vi "iscan.vi"(0 "IP adress":string="192.109.209.229", 1 "stop":bool, 2 "Channel":u8(ring)=12 items=["1", "2", "3", "4", "5", "6", "7", "8", "9", "10", "11", "12", "13", "14", "15", "16"], 3 "ISCAN Parameters":T1={"vs_initial "=TRUE, "Current_step"=0.0, "Scans"=[{" vs_initial"=FALSE, "Current_step"=0.001, "Scan_Rate"=1.0}, {" vs_initial"=FALSE, "Current_step"=-0.001, "Scan_Rate"=1.0}, {" vs_initial"=FALSE, "Current_step"=0.0, "Scan_Rate"=1.0}], "Scan_number"=2, "N_Cycles"=1, "Record_every_dI"=1e-05, "Begin_measuring_E"=0.5, "End_measuring_E"=0.75, "I_Range"=7, "E_Range"=2, "Bandwidth"=5, "em"=1, "ce"=0, "tb"=5e-05} {"tb" min=5e-05 max=1 format="%^_3e"; "ce" items=["Standard", "CE to ground"]; "End_measuring_E" min=0 max=1 format="%.2f"; "Begin_measuring_E" min=0 max=1 format="%.2f"; "Current_step" min=-150 max=150 format="%^_3e"; "N_Cycles" min=0 max=1000000; "Scan_number" min=0 max=98; "Scans"."Scan_Rate" min=0.01 max=1000 format="%^_3e"; "Scans"."Current_step" min=-150 max=150 format="%^_3e"; "E_Range" items=["±2.5V", "±5V", "±10V", "Auto"]; "Bandwidth" items=["1"=1, "2"=2, "3"=3, "4"=4, "5"=5, "6"=6, "7"=7, "8"=8, "9"=9]; "Record_every_dI" format="%^_3e"; "I_Range" items=["1pA", "1nA", "10nA", "100nA", "1µA", "10µA", "100µA", "1mA", "10mA", "100mA", "1A", "Booster"]}, 4 "Exit":bool, 5 "Start":bool, 6 "Draw":enum16{"I(Ewe)", "Ewe(t)", "I(t)"}(ring)=enum."I(t)") -> (7 "XY Graph":cluster{"Data 101":sgl[], "Data 101":sgl[]}(graph), 8 "Number of points":i32=105)   [LabVIEW 2016]
doc: "The Current scan technique (Galvanodynamic Technique) technique allows the user to perform galvanodynamic periods with different scan rates.\nIn general, in this VI, the first thing to do is to start by establishing the connection with the instrument defined by its IP adress, then load the firmware in the channel selected, get the information on the plugged channels, load protocol on a channel, start/stop the protocol, retreive data and draw the graph."
uses:
  LLB/dll_Functions.llb/ISCANParameters.ctl
panel:
  in  "Display Parameters?":bool caption="Display Parameters"
  out "DllPath":path caption="DLL Path"
  out "LibVersion":string caption="DLL Version"
  out "Device Code":i32
  out "Exit 2":bool=TRUE
  out "Data 125":sgl[][](array[numeric])=[[0.003, 0.0019739384, 6.01559e-07, 0.002076381], [0.105000004, 0.012167796, 2.1901733e-06, 0.0117511805], [0.20700002, 0.022361653, 3.975648e-06, 0.021977918], [0.30900002, 0.03255551, 5.772186e-06, 0.032090176], [0.411, 0.042749364, 7.5965745e-06, 0.042278755], [0.513, 0.052943222, 9.43279e-06, 0.052619968], [0.615, 0.06313708, 1.1011484e-05, 0.06277039], [0.717, 0.07333094, 1.3262951e-05, 0.07292081], [0.81900007, 0.08352479, 1.5135982e-05, 0.082956746], [0.92, 0.09371865, 1.6970866e-05, 0.09329796], [1.146, 0.08352479, 1.50444275e-05, 0.083796255], [1.248, 0.07333094, 1.3190472e-05, 0.07337872], [1.35, 0.06313708, 1.1359403e-05, 0.06338094], [1.4510001, 0.052943222, 9.505447e-06, 0.053039722], [1.5530001, 0.042749364, 7.704897e-06, 0.042965624], [1.6550001, 0.03255551, 5.7821057e-06, 0.03273889], [1.7570001, 0.022361653, 3.9939605e-06, 0.02243583], [1.8590001, 0.012167796, 2.2004742e-06, 0.012209094], [1.9610001, 0.0019739384, 3.9210917e-07, 0.0019060377], [2.0630002, -0.008219917, -1.42999e-06, -0.007939104], [2.1650002, -0.018413773, -3.2925293e-06, -0.01812768], [2.2670002, -0.02860763, -5.1661327e-06, -0.028087301], [2.3690002, -0.038801484, -7.0229494e-06, -0.038695633], [2.4710002, -0.048995342, -8.872135e-06, -0.048960526], [2.5730002, -0.059189197, -1.0682789e-05, -0.059149105], [2.6750002, -0.069383055, -1.2368184e-05, -0.06929952], [2.7770002, -0.07957691, -1.4145845e-05, -0.079564415], [2.8790002, -0.089770764, -1.595784e-05, -0.08963852], [2.9810002, -0.09996462, -1.7746945e-05, -0.09997973], [3.0830002, -0.11015848, -1.9597086e-05, -0.11005383], [3.1840003, -0.120352335, -2.1420525e-05, -0.1202424], [3.2860003, -0.13054618, -2.3339331e-05, -0.13024017], [3.3880002, -0.14074004, -2.5181842e-05, -0.14054324], [3.4900002, -0.1509339, -2.7039614e-05, -0.15061733], [3.5920002, -0.16112776, -2.8866867e-05, -0.16069143], [3.6940002, -0.17132162, -3.0690302e-05, -0.17118528], [3.7960002, -0.18151547, -3.246415e-05, -0.18129754], [3.8980002, -0.19170932, -3.425326e-05, -0.19167691], [4.1660004, -0.18151547, -3.2410746e-05, -0.1819081], [4.268, -0.17132162, -3.064834e-05, -0.17160504], [4.3700004, -0.16112776, -2.8840164e-05, -0.1615691], [4.472, -0.1509339, -2.6993837e-05, -0.15141869], [4.5740004, -0.14074004, -2.5170399e-05, -0.14126827], [4.676, -0.13054618, -2.3297369e-05, -0.13085073], [4.7780004, -0.120352335, -2.1454858e-05, -0.120471366], [4.88, -0.11015848, -1.9608531e-05, -0.11066438], [4.9820004, -0.09996462, -1.7731685e-05, -0.100361325], [5.084, -0.089770764, -1.5908246e-05, -0.09028722], [5.1860003, -0.07957691, -1.4138216e-05, -0.07979337], [5.288, -0.069383055, -1.23643695e-05, -0.06975743], [5.3900003, -0.059189197, -1.0510413e-05, -0.059530698], [5.491, -0.048995342, -8.728937e-06, -0.049342122], [5.5930004, -0.038801484, -6.897869e-06, -0.039191704], [5.695, -0.02860763, -5.1615543e-06, -0.029041288], [5.7970004, -0.018413773, -3.292148e-06, -0.018547434], [5.899, -0.008219917, -1.4265564e-06, -0.008549656], [6.0010004, 0.0019739384, 4.397981e-07, 0.0014481241], [6.103, 0.012167796, 2.245111e-06, 0.011636702], [6.2050004, 0.022361653, 4.0595805e-06, 0.021939758], [6.307, 0.03255551, 5.846962e-06, 0.032090176], [6.4090004, 0.042749364, 7.638159e-06, 0.04212612], [6.511, 0.052943222, 9.431646e-06, 0.05246733], [6.6130004, 0.06313708, 1.1045057e-05, 0.062579595], [6.715, 0.07333094, 1.3209546e-05, 0.07276817], [6.8170004, 0.08352479, 1.5067316e-05, 0.08303307], [6.919, 0.09371865, 1.690983e-05, 0.09318349], [7.1440005, 0.08352479, 1.5128351e-05, 0.08364362], [7.2460003, 0.07333094, 1.3301099e-05, 0.0733024], [7.3480005, 0.06313708, 1.1408995e-05, 0.06338094], [7.4490004, 0.052943222, 9.520706e-06, 0.053039726], [7.5510006, 0.042749364, 7.704897e-06, 0.042316914], [7.6530004, 0.03255551, 5.7290754e-06, 0.032624412], [7.7550006, 0.022361653, 3.9203287e-06, 0.02262663], [7.8570004, 0.012167796, 2.1073854e-06, 0.012056456], [7.9590006, 0.0019739384, 3.3221184e-07, 0.0022876323], [8.061001, -0.008219917, -1.4410538e-06, -0.007900944], [8.163, -0.018413773, -3.2478924e-06, -0.017975042], [8.265, -0.02860763, -5.089448e-06, -0.028316258], [8.367001, -0.038801484, -6.929479e-06, -0.038504835], [8.469001, -0.048995342, -8.814146e-06, -0.04869341], [8.571, -0.059189197, -1.0662569e-05, -0.059263583], [8.673, -0.069383055, -1.2417775e-05, -0.06933768], [8.775001, -0.07957691, -1.42297695e-05, -0.079144664], [8.877001, -0.089770764, -1.6053207e-05, -0.0893714], [8.979, -0.09996462, -1.7861388e-05, -0.09982709], [9.081, -0.11015848, -1.9642863e-05, -0.10990119], [9.182, -0.120352335, -2.1462487e-05, -0.12020425], [9.284, -0.13054618, -2.3247778e-05, -0.13043097], [9.386001, -0.14074004, -2.5071215e-05, -0.14046691], [9.488001, -0.1509339, -2.6944244e-05, -0.15084629], [9.59, -0.16112776, -2.8832534e-05, -0.16084407], [9.692, -0.17132162, -3.0682673e-05, -0.17129977], [9.794001, -0.18151547, -3.2525186e-05, -0.18110675], [9.896001, -0.19170932, -3.435244e-05, -0.19156244], [10.1640005, -0.18151547, -3.2357337e-05, -0.18206073], [10.266001, -0.17132162, -3.0552972e-05, -0.1716432], [10.368, -0.16112776, -2.8763869e-05, -0.16137831], [10.47, -0.1509339, -2.6936617e-05, -0.15138052], [10.5720005, -0.14074004, -2.5143696e-05, -0.14138275], [10.674001, -0.13054618, -2.3377479e-05, -0.1306981], [10.776001, -0.120352335, -2.1515893e-05, -0.12066216], [10.878, -0.11015848, -1.9719157e-05, -0.11047359], [10.9800005, -0.09996462, -1.780798e-05, -0.100513965], [11.082001, -0.089770764, -1.5946394e-05, -0.09021091], [11.184001, -0.07957691, -1.4088625e-05, -0.079869695]] format="%.2f"
  # "Instructions:\nBefore running the VI you must type a valid IP adress that corresponds to the instrument.Then press the Run button to execute this VI.\nWhile this VI is running, choose the available channel, enter the ISCAN parameters or keep the default values, then press the button start to begin the experience.\nChoose the waveform to draw (Ewe(t) or I(t) or I(Ewe) or Ec(t). You can stop the measure if you press the stop button and exit the execution if you press the exit button."
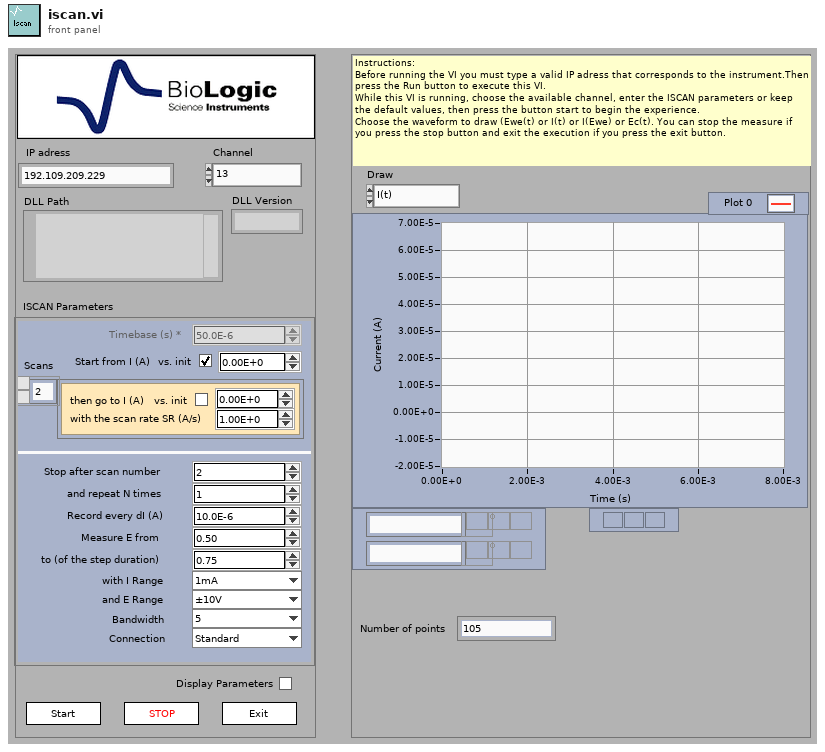
[diagram p1: front panel]
types:
  T1 = typedef "ISCANParameters.ctl" = cluster{"vs_initial ":bool, "Current_step":sgl, "Scans":cluster{" vs_initial":bool, "Current_step":sgl, "Scan_Rate":sgl}[], "Scan_number":i32, "N_Cycles":i32, "Record_every_dI":sgl, "Begin_measuring_E":sgl, "End_measuring_E":sgl, "I_Range":u16, "E_Range":u16, "Bandwidth":u16, "em":u16, "ce":u16, "tb":sgl}
  T2 = cluster{"LibVersion":string, "StringLength":u32, "DllPath":path}
  T3 = cluster{"Channel":i32, "BoardVersion":i32, "BoardSerialCode":i32, "FirmwareCode":i32, "FirmwareVersion":i32, "XilinxVersion":i32, "AmpCode":i32, "NbAmp":i32, "LcBoard":i32, "Zboard":i32, "MuxBoard":i32, "GPRAboard":i32, "MemSize":i32, "MemFilled":i32, "state":i32, "MaxIRange":i32, "MinIRange":i32, "MaxBandwidth":i32, "NbOfTechniques":i32}
  T4 = typedef "TechniqueParameters.ctl" = cluster{"String Label":string, "Type":i32, "Valeur":i32, "Index":i32}
  T5 = cluster{"string before end tag":string, i32, i32, i32}[]
  T6 = cluster{"IRQskipped":i32, "NbRaws":i32, "NbCols":i32, "Technique Index":i32, "TechniqueID":i32, "PrcessIndex":i32, "loop":i32, "StartTime":dbl, "MuxPad":i32}
  T7 = cluster{"State":i32, "MemFilled":i32, "TimeBase":sgl, " Ewe":sgl, " EweRangeMin":sgl, " EweRangeMax":sgl, "Ece":sgl, "EceRangeMin":sgl, "EceRangeMax":sgl, "Eoverflow":i32, "I":sgl, "IRange":i32, "Ioverflow":i32, "ElapsedTime":sgl, "Freq":sgl, "Rcomp":sgl, "Saturation":sgl, "OptErr":i32, "OptPos":i32}
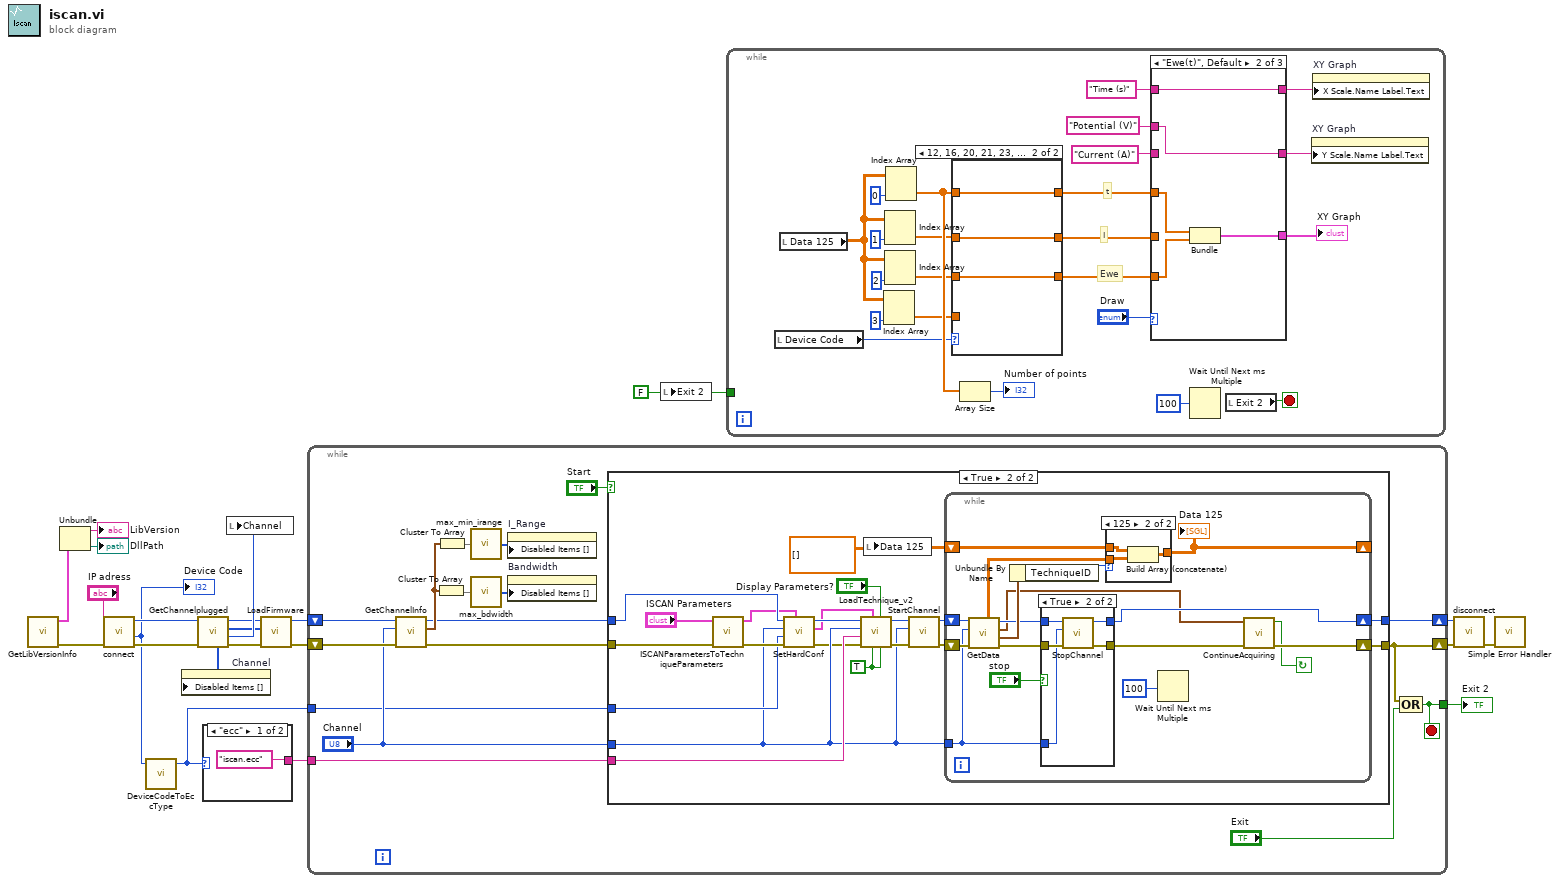
[diagram p0: block diagram]
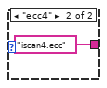
[diagram p2: hidden frame]
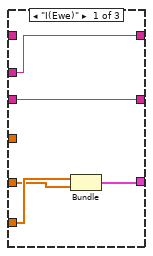
[diagram p4: hidden frame]
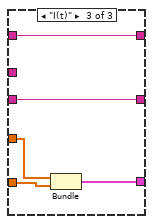
[diagram p5: hidden frame]
diagram:
  w20 = FALSE ("Exit 2")
  n1 = call "GetLibVersionInfo.vi"() -> ("error out"=w1:errorcluster, "LibInfo"=w4:T2)  [unwired: 10 in]
  n2 = Unbundle(w4) -> ("LibVersion"=→"LibVersion":string, "DllPath"=→"DllPath":path)  [unwired: 1 out]
  n3 = call "connect.vi"("error in (no error)"=w1, "IP"="IP adress") -> ("error out"=w16:errorcluster, "Device Code"=w10:i32, "ID Out"=w17:i32)  [unwired: 6 in, 1 out]
  "Device Code" <- w10
  n4 = call "DeviceCodeToEccType.vi"("Device Code"=w10) -> ("EccType"=w5:enum16{"ecc", "ecc4"})  [unwired: 4 in]
  n5 = call "GetChannelplugged.vi"("error in (no error)"=w16, "ID In"=w17) -> ("error out"=w15:errorcluster, "FirstPluggedChannel"=w18:u8, "PluggedChannels"=w13:u8[], "DisabledChannels"=w14:i32[])  [unwired: 5 in, 1 out]
  n6 = property on="Channel" class="Ring (strict)"("Disabled Items []"=w14) -> ()  [unwired: 2 in, 2 out]
  n7 = case shown="\"ecc\"" w5 {
    tunnel: ["iscan.ecc" ("FName") "iscan4.ecc" ("FName4")] -> w9
    frame "ecc" {
    }
    frame "ecc4" {
    }
  }
  n8 = local write "Channel"(w18) -> ()
  n9 = call "LoadFirmware.vi"("error in (no error)"=w15, "Channels"=w13, "ID In"=w17) -> ("error out"=w12:errorcluster)  [unwired: 6 in, 2 out]
  n10 = while {
    shift-right: [w26] -> w11
    shift-left: w12 -> [w33]
    tunnel: w9 -> [w28]
    shift-right: [w27] -> w8
    shift-left: w17 -> [w34]
    tunnel: [w24] -> w7
    tunnel: w5 -> [w23]
    stop <- w24 stop-if-true
    n11 = call "GetChannelInfo.vi"("error in (no error)"=w33, "Channel"="Channel", "ID"=w34) -> ("error out"=w31:errorcluster, "Channel information"=w30:T3, "ID Out"=w29:i32)  [unwired: 6 in]
    n12 = Cluster To Array(cluster=w30) -> (array=w37:i32[])
    n13 = Cluster To Array(cluster=w30) -> (array=w38:i32[])
    n14 = call "max_min_irange.vi"("resources"=w38) -> ("disabled ranges"=w35:i32[])
    n15 = call "max_bdwidth.vi"("resources"=w37) -> ("disabled ranges"=w36:i32[])
    n16 = property on="I_Range" class="Ring (strict)"("Disabled Items []"=w35) -> ()  [unwired: 2 in, 2 out]
    n17 = property on="Bandwidth" class="Ring (strict)"("Disabled Items []"=w36) -> ()  [unwired: 2 in, 2 out]
    n18 = case shown="True" "Start" {
      tunnel: "Channel" -> [_ w44]
      tunnel: [w41 w61] -> w26
      tunnel: w31 -> [w41 w51]
      tunnel: [w40 w52] -> w27
      tunnel: w29 -> [w40 w49]
      tunnel: w28 -> [_ w57]
      tunnel: w23 -> [_ w45]
      frame False {
      }
      frame True {
        w58 = TRUE ("First Protocol")
        w60 = sgl[][] []
        n19 = call "ISCANParametersToTechniqueParameters.vi"("error in (no error)"=w51, "ISCAN Parameters"="ISCAN Parameters") -> ("error out"=w50:errorcluster, "TechniqueParameters"=w46:T4[])  [unwired: 8 in]
        n20 = call "SetHardConf.vi"("Params Values"=w46, "error in (no error)"=w50, "EccType"=w45, "Channel"=w44, "ID In"=w49) -> ("error out"=w43:errorcluster, "Params Values Trimed"=w47:T5, "ID Out"=w48:i32)  [unwired: 4 in]
        n21 = call "LoadTechnique_v2.vi"("Last Protocol"=w58, "Display Parameters?"="Display Parameters?", "First Protocol"=w58, "TechniqueParameters"=w47, "error in (no error)"=w43, "FName"=w57, "Selected Channel"=w44, "ID In"=w48) -> ("error out"=w56:errorcluster, "ID  Out"=w55:i32)  [unwired: 2 in]
        n22 = local write "Data 125"(w60) -> ()
        n23 = call "StartChannel.vi"("error in (no error)"=w56, "Channel"=w44, "ID In"=w55) -> ("error out"=w54:errorcluster, "ID Out"=w53:i32)  [unwired: 7 in]
        n24 = while {
          shift-right: [w64] -> w61
          shift-left: w54 -> [w78]
          shift-right: [w75] -> _
          shift-left: w60 -> [w76]
          shift-right: [w67] -> w52
          shift-left: w53 -> [w70]
          tunnel: w44 -> [w66]
          stop <- w62 continue-if-true
          n25 = call "GetData.vi"("error in (no error)"=w78, "Channel"=w66, "ID In"=w70) -> ("error out"=w69:errorcluster, "Data information"=w72:T6, "Current values"=w65:T7, "ID Out"=w68:i32, "Data"=w71:dbl[][])  [unwired: 4 in]
          n26 = Unbundle By Name(w72) -> ("TechniqueID"=w73:i32)
          n27 = case shown="True" "stop" {
            tunnel: [w79 w85] -> w63
            tunnel: w69 -> [w79 w84]
            tunnel: w68 -> [w80 w83]
            tunnel: [w80 w82] -> w67
            tunnel: w66 -> [_ w81]
            frame False {
            }
            frame True {
              n28 = call "StopChannel.vi"("error in (no error)"=w84, "Channel"=w81, "ID In"=w83) -> ("error out"=w85:errorcluster, "ID Out"=w82:i32)  [unwired: 7 in]
            }
          }
          n29 = case shown="125" w73 {
            tunnel: w76 -> [w86 w89]
            tunnel: [w86 w88] -> w75
            tunnel: w71 -> [_ w87]
            frame 0, Default {
            }
            frame 125 {
              n30 = Build Array (concatenate)(w89, w87) -> (w88:dbl[][])
            }
          }
          "Data 125" <- w75
          n31 = Wait Until Next ms Multiple(millisecond multiple=u32 100) -> ()  [unwired: 1 out]
          n32 = call "ContinueAcquiring.vi"("error in"=w63, "Current values"=w65) -> ("error out"=w64:errorcluster, "ContinueAcquiring?"=w62:bool)  [unwired: 8 in]
        }
      }
    }
    n33 = Compound Arithmetic op=OR(w26, "Exit") -> (w24:bool)
  }
  "Exit 2" <- w7
  n34 = local write "Exit 2"(w20) -> ()
  n35 = while {
    tunnel: w20 -> [_]
    stop <- w111 stop-if-true
    # "Ewe"
    # "I"
    # "t"
    n36 = local read "Device Code"() -> (w90:i32)
    n37 = local read "Data 125"() -> (w99:sgl[][])
    n38 = Index Array(array=w99, index (col)=3 ("Index")) -> (element=w92:sgl[])  [unwired: 1 in]
    n39 = Index Array(array=w99, index (col)=1 ("Index")) -> (element=w95:sgl[])  [unwired: 1 in]
    n40 = Index Array(array=w99, index (col)=2 ("Index")) -> (element=w94:sgl[])  [unwired: 1 in]
    n41 = Index Array(array=w99, index (col)=0 ("Index")) -> (element=w97:sgl[])  [unwired: 1 in]
    n42 = case shown="12, 16, 20, 21, 23, 27" w90 {
      tunnel: w97 -> [w115 w118]
      tunnel: [w115 w118] -> w96
      tunnel: w95 -> [_ w117]
      tunnel: w94 -> [w114 w116]
      tunnel: [w114 w117] -> w93
      tunnel: w92 -> [w113 _]
      tunnel: [w113 w116] -> w91
      frame 0, Default {
      }
      frame 12, 16, 20, 21, 23, 27 {
      }
    }
    n43 = Array Size(array=w97) -> (size(s)=→"Number of points":i32)
    n44 = case shown="\"Ewe(t)\", Default" "Draw" {
      tunnel: w96 -> [_ w128 w133]
      tunnel: w93 -> [w120 _ w132]
      tunnel: [w119 w124 w129] -> w98
      tunnel: "Potential (V)" ("Y Scale.Name Label.Text") -> [w123 w127 _]
      tunnel: "Current (A)" ("Y Scale.Name Label.Text") -> [w122 _ w131]
      tunnel: [w122 w127 w131] -> w103
      tunnel: [w123 w126 w130] -> w102
      tunnel: "Time (s)" ("Y Scale.Name Label.Text") -> [_ w126 w130]
      tunnel: w91 -> [w121 w125 _]
      frame "I(Ewe)" {
        n45 = Bundle("Data 125"=w121, "Data 125"=w120) -> (w119:cluster{"Data 125":sgl[], "Data 125":sgl[]})  [unwired: 1 in]
      }
      frame "Ewe(t)", Default {
        n46 = Bundle("Data 125"=w128, "Data 125"=w125) -> (w124:cluster{"Data 125":sgl[], "Data 125":sgl[]})  [unwired: 1 in]
      }
      frame "I(t)" {
        n47 = Bundle("Data 125"=w133, "Data 125"=w132) -> (w129:cluster{"Data 125":sgl[], "Data 125":sgl[]})  [unwired: 1 in]
      }
    }
    "XY Graph" <- w98
    n48 = Wait Until Next ms Multiple(millisecond multiple=u32 100) -> ()  [unwired: 1 out]
    n49 = local read "Exit 2"() -> (w111:bool)
    n50 = property on="XY Graph" class="XYGraph (strict)"("Y Scale.Name Label.Text"=w103) -> ()  [unwired: 2 in, 2 out]
    n51 = property on="XY Graph" class="XYGraph (strict)"("X Scale.Name Label.Text"=w102) -> ()  [unwired: 2 in, 2 out]
  }
  n52 = call "disconnect.vi"("error in (no error)"=w11, "ID In"=w8) -> ("error out"=w6:errorcluster)  [unwired: 9 in]
  n53 = call <vilib>:"Simple Error Handler.vi"("error in (no error)"=w6) -> ()  [unwired: 4 in, 5 out]
